vi "CalcStrafeAngles.vi"(9 "Speed":dbl, 10 "Y":dbl, 11 "X":dbl) -> (3 "StrafeAngle":dbl)   [LabVIEW 2017]
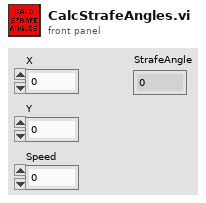
[diagram p1: front panel]
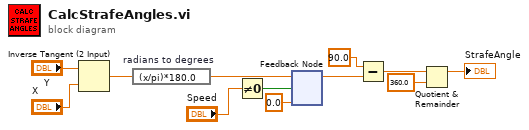
[diagram p0: block diagram]
diagram:
  n1 = Inverse Tangent (2 Input)(1:"X", 2:"Y") -> (0:w12:dbl)
  n2 = expression code="(x/pi)*180.0" "radians to degrees"(w12) -> (w11:dbl)
  n3 = Not Equal To 0?(x="Speed") -> (x != 0?=w10:bool)
  n4 = feedback #1(0.0) -> (w5:dbl)
  n5 = feedback-in #1(w11, w10) -> ()
  n6 = Subtract(x=90.0, y=w5) -> (x-y=w8:dbl)
  n7 = Quotient & Remainder(x=w8, y=360.0) -> (x-y*floor(x/y)=→"StrafeAngle":dbl)  [unwired: 1 out]
